vi "Set Name.vi"(8 "error in (no error)":errorcluster, 10 "Name":string, 11 "LVType.lvclass in":refnum<class "LVType.lvclass">) -> (0 "error out":errorcluster, 3 "LVType.lvclass out":refnum<class "LVType.lvclass">)   [LabVIEW 2020, in "LVDataTypes.lvlib" / "LVType.lvclass"]
uses:
  <vilib>/AppBuilder/Engine/WebServiceDescription/LVDataTypes/LVType/LVType.lvclass
  <vilib>/AppBuilder/Engine/WebServiceDescription/LVDataTypes/LVType/LVType.lvclass/LVType.ctl
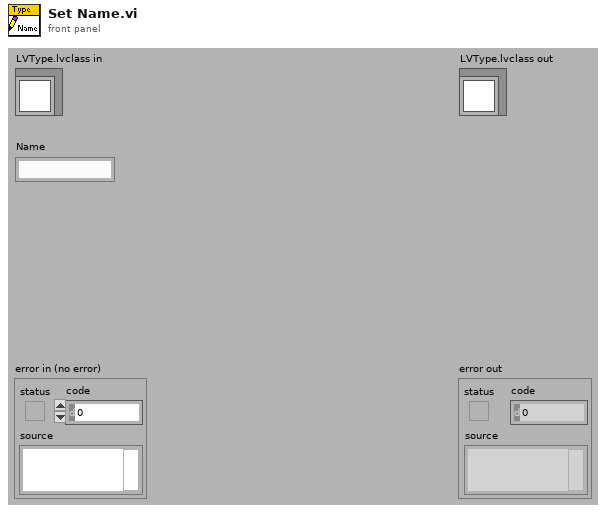
[diagram p1: front panel]
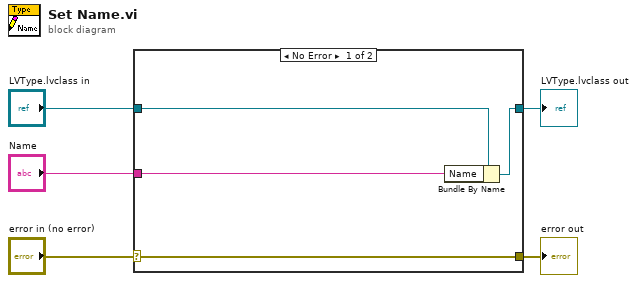
[diagram p0: block diagram]
diagram:
  n1 = case shown="No Error" "error in (no error)" {
    selector: "error in (no error)" -> [w9 w10]
    tunnel: [w9 w10] -> w4
    tunnel: [w7 w11] -> w2
    tunnel: "LVType.lvclass in" -> [w8 w11]
    tunnel: "Name" -> [w6 _]
    frame No Error {
      n2 = Bundle By Name(cluster=w8, "Name"=w6) -> (w7:refnum<class "LVType.lvclass">)
    }
    frame Error {
    }
  }
  "error out" <- w4
  "LVType.lvclass out" <- w2
